vi "modulation - Copy.vi"() -> ()   [LabVIEW 2018]
uses:
  <vilib>/express/express arith-compare/Formula/XNode/ExpressFormulaBlockNode.xnode
panel:
  in  "Amplitude 2":dbl=1.0 caption="Amplitude"
  in  "Amplitude":dbl=1.0
  out "Modulated Wave":dbl(graph)
  out "Carrier Signal":dynamicdata(graph)
  out "Message signal":dynamicdata(graph)
  in  "Modulation index":dbl(knob) scale=0.0..100.0
  in  "Carrier Frequency":dbl(knob) scale=0.0..100.0
  in  "Message frequency":dbl(knob) scale=0.0..100.0
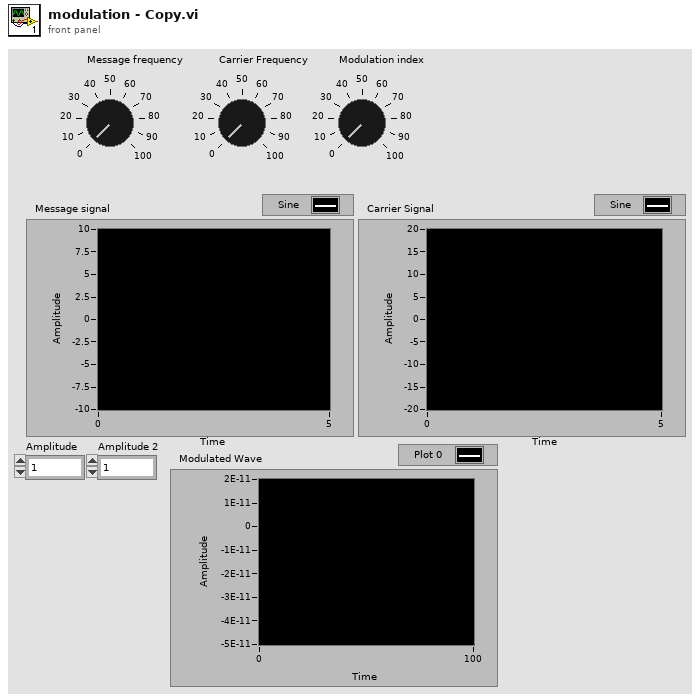
[diagram p1: front panel]
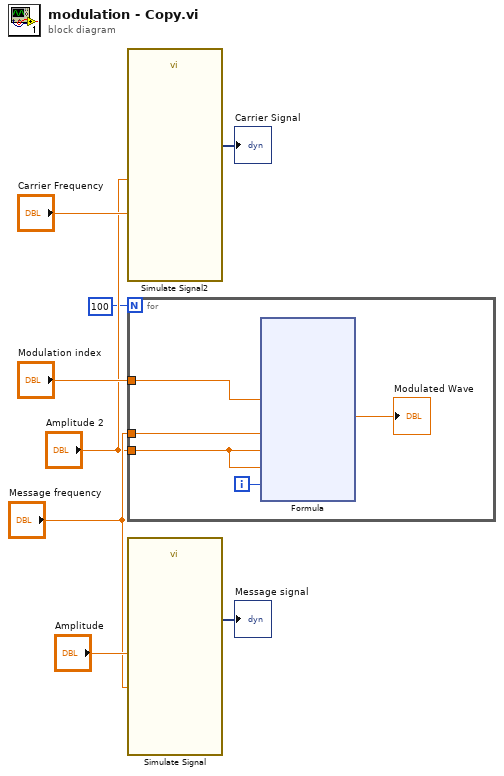
[diagram p0: block diagram]
diagram:
  n1 = call "Simulate Signal2"("Frequency"="Carrier Frequency", "Amplitude"="Amplitude 2") -> ("Sine"=→"Carrier Signal":dynamicdata)  [unwired: 12 in, 1 out]
  n2 = for {
    N: 100 -> [_]
    tunnel: "Modulation index" -> [w12]
    tunnel: "Message frequency" -> [w11]
    tunnel: "Amplitude 2" -> [w10]
    i -> [w9]
    n3 = xnode "Formula"("K"=w12, "Fm"=w11, "Fc"=w10, "Ac"=w10, "t"=w9) -> ("Result"=→"Modulated Wave":dbl)  [unwired: 1 in, 1 out]
  }
  n4 = call "Simulate Signal"("Frequency"="Message frequency", "Amplitude"="Amplitude") -> ("Sine"=→"Message signal":dynamicdata)  [unwired: 12 in, 1 out]
